vi "Add_xls.vi"   [LabVIEW 2010]
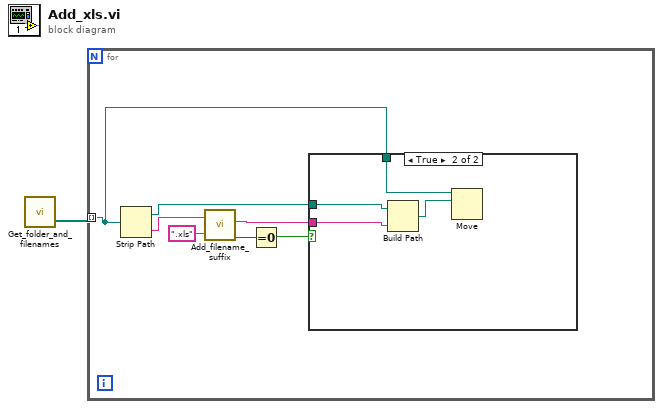
[diagram p0: block diagram]
diagram:
  n1 = call "Get_folder_and_filenames.vi"() -> ("Files"=w1:path[])  [unwired: 1 in, 1 out]
  n2 = for {
    tunnel: w1 -> [w8] mode=indexing
    n3 = Strip Path(path=w8) -> (stripped path=w3:path, name=w7:string)
    n4 = call "Add_filename_suffix.vi"("Filename"=w7, "Suffix to add"=".xls") -> ("Filename out"=w2:string, "Extension length"=w5:i32)  [unwired: 2 out]
    n5 = Equal To 0?(x=w5) -> (x = 0?=w4:bool)
    n6 = case shown="True" w4 {
      tunnel: w8 -> [_ w12]
      tunnel: w3 -> [_ w10]
      tunnel: w2 -> [_ w9]
      frame False {
      }
      frame True {
        n7 = Build Path(base path=w10, name or relative path=w9) -> (appended path=w11:path)
        n8 = Move(source path=w12, 10:w11) -> ()  [unwired: 3 in, 3 out]
      }
    }
  }
